vi "PeakDetect.vi"() -> ()   [LabVIEW 2015]
uses:
  <vilib>/Analysis/NI_AALPro.lvlib
panel:
  in  "minimumPeakWidth":dbl format="%#_13g"
  in  "minPeakHeightFraction":dbl format="%#_13g"
  in  "MinimumPeakWidth":dbl=0.8
  in  "Data Path":path=path "D:/GITRepositories/Ionics/GitHub/EH-QfirmwareServer/firmware-server/Sniffer.900/Server/PeakDetection/Q1 PPG Pos IonSniffer-140926.txt"
  in  "Search Window":dbl=0.8
  in  "RefMass":dbl=1778.3
  in  "threshold":dbl=1000.0
  out "XY Graph":cluster{"X":dbl, "Y":dbl}[](graph)
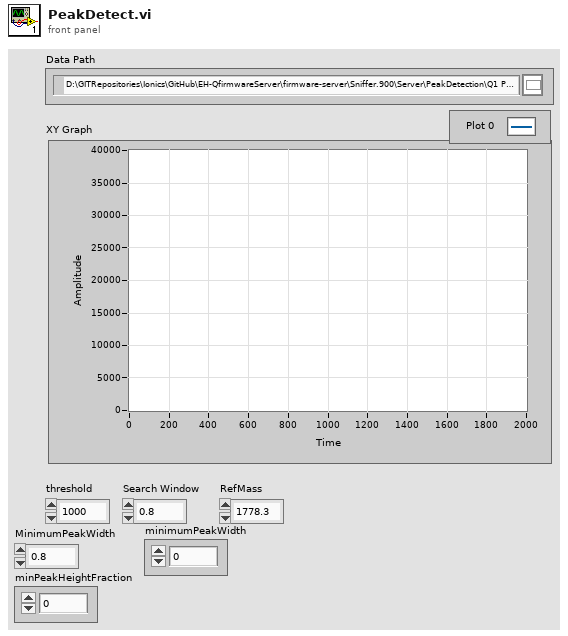
[diagram p1: front panel]
types:
  T1 = typedef "PeakInfoPresenter.ctl" = cluster{"PeakHeight":dbl, "PeakHeightIndex":dbl, "StartIndex":dbl, "EndIndex":dbl, "PeakValue":dbl, "StartValue":dbl, "EndValue":dbl}
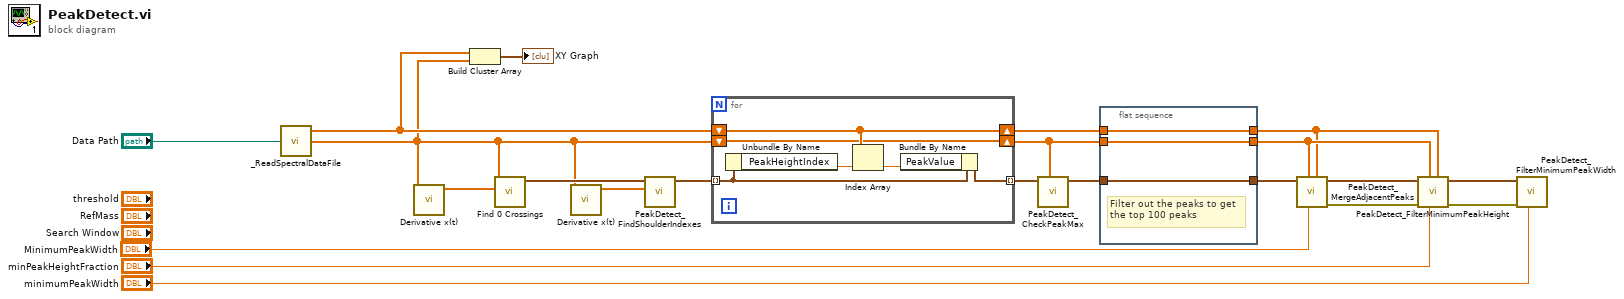
[diagram p0: block diagram]
diagram:
  n1 = call "_ReadSpectralDataFile.vi"("file path (dialog if empty)"="Data Path") -> ("Y"=w15:dbl[], "X"=w16:dbl[])  [unwired: 1 out]
  n2 = call <vilib>:"Derivative x(t).vi"("X"=w15) -> ("dX/dt"=w20:dbl[])  [unwired: 9 in, 1 out]
  n3 = Build Cluster Array(w16, w15) -> (→"XY Graph":cluster{dbl, dbl}[])
  n4 = call "Find 0 Crossings.vi"("dX/dt"=w20, "Intensities"=w15) -> ("Peaks Info"=w19:T1[])  [unwired: 8 in, 1 out]
  n5 = call <vilib>:"Derivative x(t).vi"("X"=w15) -> ("dX/dt"=w18:dbl[])  [unwired: 9 in, 1 out]
  n6 = call "PeakDetect_FindShoulderIndexes.vi"("2nd Deriv"=w18, "Peaks Info"=w19) -> ("Array"=w17:T1[])  [unwired: 9 in]
  n7 = for {
    tunnel: w17 -> [w28] mode=indexing
    tunnel: [w27] -> w14 mode=indexing
    shift-right: [w24] -> w11
    shift-left: w16 -> [w24]
    shift-right: [w23] -> w12
    shift-left: w15 -> [w23]
    n8 = Unbundle By Name(w28) -> ("PeakHeightIndex"=w26:dbl)
    n9 = Index Array(array=w24, index=w26) -> (element=w25:dbl)
    n10 = Bundle By Name(cluster=w28, "PeakValue"=w25) -> (w27:T1)
  }
  n11 = call "PeakDetect_CheckPeakMax.vi"("Intensities"=w12, "Peak Presenter"=w14) -> ("Peak Presenter 2"=w13:T1[])  [unwired: 9 in]
  n12 = flat-sequence {
    tunnel: w13 -> [w31]
    tunnel: w12 -> [w30]
    tunnel: w11 -> [w29]
    tunnel: [w31] -> w10
    tunnel: [w30] -> w6
    tunnel: [w29] -> w5
    frame #0 {
      # "Filter out the peaks to get\nthe top 100 peaks"
    }
  }
  n13 = call "PeakDetect_MergeAdjacentPeaks.vi"("Masses"=w5, "MinimumPeakWidth"="MinimumPeakWidth", "Intensities"=w6, "Peak Info In"=w10) -> ("Error Out"=w7:errorcluster, "Peak Info Out"=w8:T1[])  [unwired: 6 in]
  n14 = call "PeakDetect_FilterMinimumPeakHeight.vi"("Masses"=w5, "minPeakHeightFraction"="minPeakHeightFraction", "Intensities"=w6, "Error In"=w7, "Peak Info In"=w8) -> ("Error Out"=w3:errorcluster, "Peak Info Out"=w2:T1[])  [unwired: 5 in]
  n15 = call "PeakDetect_FilterMinimumPeakWidth.vi"("minimumPeakWidth"="minimumPeakWidth", "Error In"=w3, "Peak Info In"=w2) -> ()  [unwired: 7 in, 2 out]
